vi "UpdateThicknessIndicators.vi"(9 "Lens thickness left":dbl, 10 "Lens thickness right":dbl, 11 "Lens thickness average":dbl) -> ()   [LabVIEW 2013]
uses:
  Global.vi
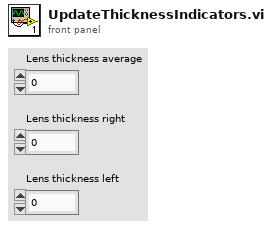
[diagram p1: front panel]
types:
  T1 = cluster{"Lens thickness left":refnum<vi>, "Lens thickness right":refnum<vi>, "Measured thickness":refnum<vi>}
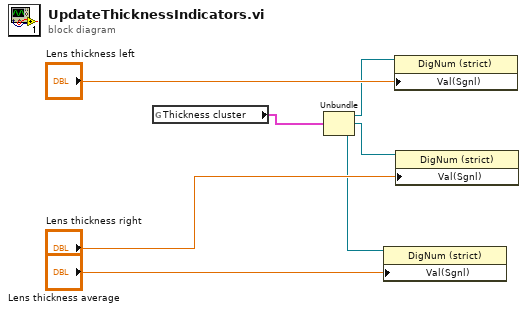
[diagram p0: block diagram]
diagram:
  n1 = global read "Global.vi" "Thickness cluster"() -> (w1:T1)
  n2 = Unbundle(w1) -> ("Lens thickness left"=w2:refnum<vi>, "Lens thickness right"=w3:refnum<vi>, "Measured thickness"=w4:refnum<vi>)
  n3 = property class="DigNum (strict)"(reference=w4, "Val(Sgnl)"="Lens thickness average") -> ()  [unwired: 1 in, 2 out]
  n4 = property class="DigNum (strict)"(reference=w2, "Val(Sgnl)"="Lens thickness left") -> ()  [unwired: 1 in, 2 out]
  n5 = property class="DigNum (strict)"(reference=w3, "Val(Sgnl)"="Lens thickness right") -> ()  [unwired: 1 in, 2 out]
